vi "Generate Next File Name.vi"(11 "Zscan State":T2) -> (3 "String":string)   [LabVIEW 2013, in "Automation.lvlib"]
uses:
  Automation.lvlib
  Zscan Settings.ctl
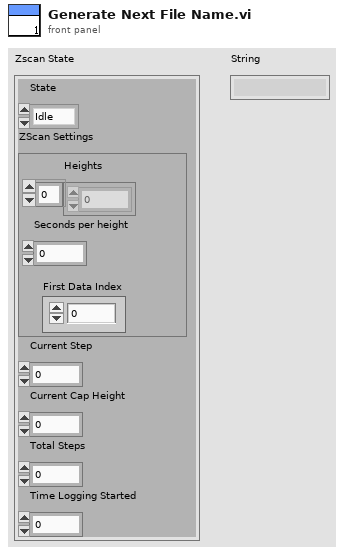
[diagram p1: front panel]
types:
  T1 = typedef "Automation.lvlib/Zscan Settings.ctl" = cluster{"Heights":dbl[], "Seconds per height":i32, "First Data Index":i32}
  T2 = cluster{"State":enum16{"Idle", "Waiting for lock", "Waiting for acquisition"}, "ZScan Settings":T1, "Current Step":i32, "Current Cap Height":dbl, "Total Steps":i32, "Time Logging Started":dbl}
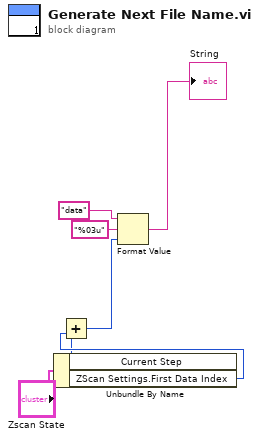
[diagram p0: block diagram]
diagram:
  n1 = Unbundle By Name("Zscan State") -> ("Current Step"=w6:i32, "ZScan Settings.First Data Index"=w7:i32)
  n2 = Add(x=w6, y=w7) -> (x+y=w3:i32)
  n3 = Format Value(string ("")="data" ("string"), format string="%03u", value (0)=w3) -> (output string=→"String":string)
